vi "WebView2 Droplet.vi"() -> ()   [LabVIEW 2020, in "WebView2.lvlib"]
uses:
  WebView2.lvlib
  C:/Users/Simon/Documents/GitHub/LV-WebView2/Source/Libs/Microsoft.Web.WebView2.WinForms.dll
  Libs/Microsoft.Web.WebView2.WinForms.dll
  WebView2 Control Object/WebView2 Control.lvclass
panel:
  in  "WebView2":refnum<k24>(container)
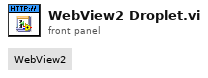
[diagram p1: front panel]
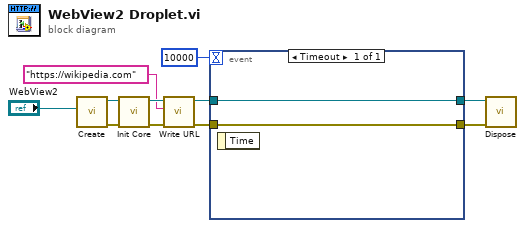
[diagram p0: block diagram]
diagram:
  n1 = call "Create.vi"("WebView2 Control"="WebView2") -> ("error out"=w10:errorcluster, "WebView2 Control out"=w8:refnum<class "WebView2 Control.lvclass">)  [unwired: 9 in]
  n2 = call "Init Core.vi"("error in (no error)"=w10, "WebView2 Control in"=w8) -> ("error out"=w9:errorcluster, "WebView2 Control out"=w7:refnum<class "WebView2 Control.lvclass">)  [unwired: 8 in]
  n3 = call "Write URL.vi"("error in (no error)"=w9, "uri"="https://wikipedia.com", "WebView2 Control in"=w7) -> ("error out"=w2:errorcluster, "WebView2 Control out"=w4:refnum<class "WebView2 Control.lvclass">)  [unwired: 7 in]
  n4 = event shown="[0] Timeout" {
    selector: _ -> [_]
    dyn-events: _ -> [_]
    timeout: 10000 -> [_]
    tunnel: [w13] -> w5
    tunnel: w4 -> [w13]
    tunnel: [w12] -> w3
    tunnel: w2 -> [w12]
    event Timeout {
      n5 = event-data() -> ()  [unwired: 1 in, 1 out]
    }
  }
  n6 = call "Dispose.vi"("error in (no error)"=w3, "WebView2 Control in"=w5) -> ()  [unwired: 9 in, 1 out]
